vi "push-strlist-test.vi"() -> ()   [LabVIEW 2019]
panel:
  in  "停止 2":bool
  in  "停止":bool
  in  "string":string
  in  "target-list":string[](array[string])
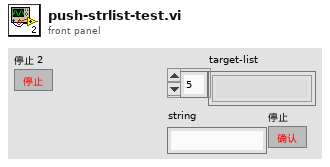
[diagram p1: front panel]
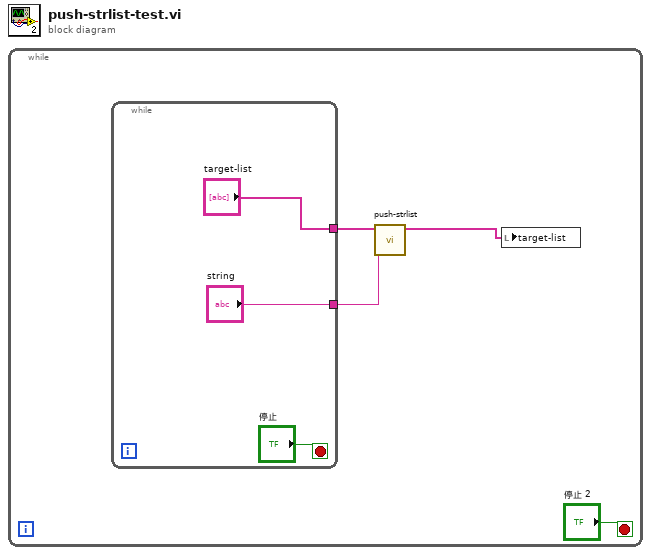
[diagram p0: block diagram]
diagram:
  n1 = while {
    stop <- "停止 2" stop-if-true
    n2 = while {
      tunnel: ["target-list"] -> w4
      tunnel: ["string"] -> w3
      stop <- "停止" stop-if-true
    }
    n3 = call "push-strlist.vi"("string"=w3, "target-list"=w4) -> ("output"=w2:string[])  [unwired: 9 in]
    n4 = local write "target-list"(w2) -> ()
  }
